vi "Network Steam Connect.vi"(6 "Timeout(ms)":i32=500, 8 "error in (no error)":errorcluster, 11 "Model in":refnum<class "Model.lvclass">) -> (0 "error out":errorcluster, 2 "Connected?":bool, 3 "Model out":refnum<class "Model.lvclass">)   [LabVIEW 2021, in "Model.lvlib" / "Model.lvclass"]
uses:
  Model.lvclass
  Model.lvclass/Model.ctl
  <userlib>/John_Lib/Network_Streams_Connection/NetworkConnection.lvclass
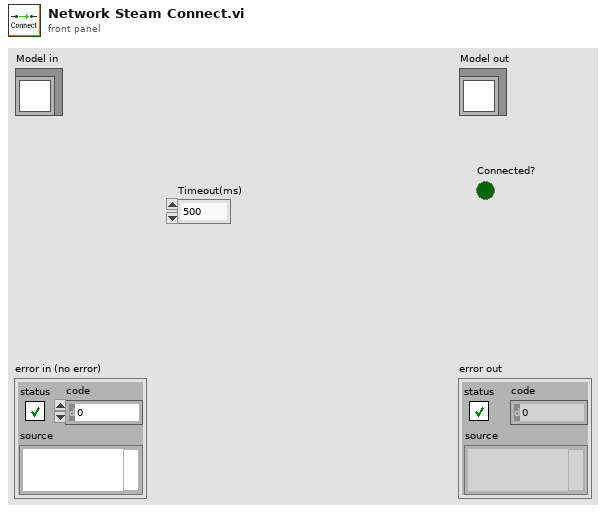
[diagram p1: front panel]
types:
  T1 = typedef "Model.lvlib/Model.lvclass/DVR.ctl" = cluster{"JKI_Network_Streams":refnum<class "NetworkConnection.lvclass">}
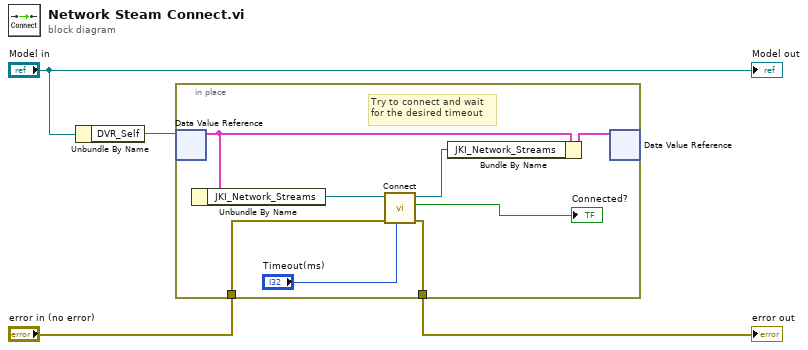
[diagram p0: block diagram]
diagram:
  n1 = Unbundle By Name("Model in") -> ("DVR_Self"=w3:refnum<data-value>)
  n2 = in-place {
    in-place-border: [w6] -> w2
    in-place-border: "error in (no error)" -> [w5]
    # "Try to connect and wait\nfor the desired timeout"
    n3 = in-place-dvr #1(w3) -> (w11:T1)  [unwired: 1 out]
    n4 = Unbundle By Name(w11) -> ("JKI_Network_Streams"=w10:refnum<class "NetworkConnection.lvclass">)
    n5 = call <userlib>:"Connect.vi"("Timeout(ms)"="Timeout(ms)", "error in (no error)"=w5, "NetworkConnection in"=w10) -> ("error out"=w6:errorcluster, "Connected?"=→"Connected?":bool, "NetworkConnection out"=w8:refnum<class "NetworkConnection.lvclass">)  [unwired: 6 in]
    n6 = Bundle By Name(cluster=w11, "JKI_Network_Streams"=w8) -> (w9:T1)
    n7 = in-place-dvr #1(w9) -> ()  [unwired: 2 out]
  }
  "error out" <- w2
  "Model out" <- "Model in"
